vi "CheckStatus.vi"(0 "VISA resource name":refnum<visa-resource-name>, 3 "error in (no error)":errorcluster) -> (1 "Idle":bool, 4 "Target Reached":bool, 5 "VISA resource name out":refnum<visa-resource-name>, 6 "Infusing":bool, 7 "Withdrawing":bool, 8 "error out":errorcluster)   [LabVIEW 2018]
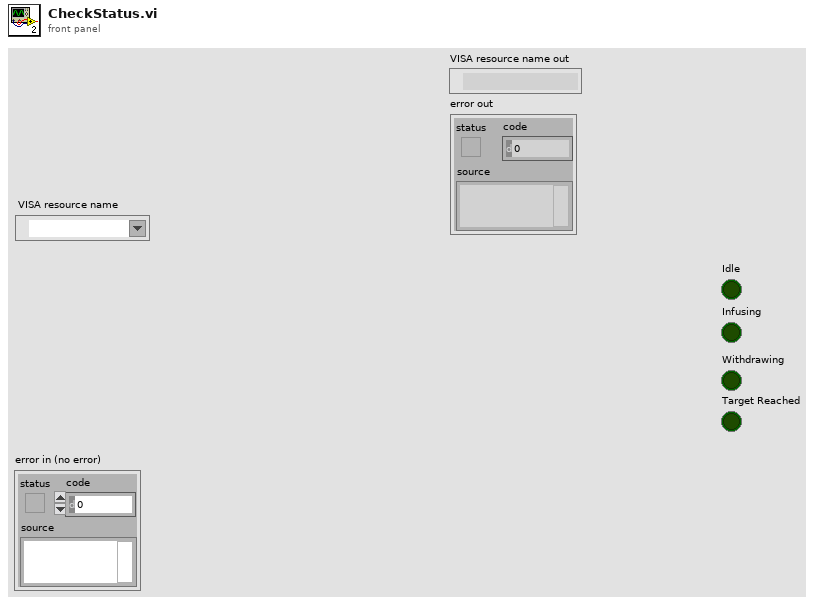
[diagram p1: front panel]
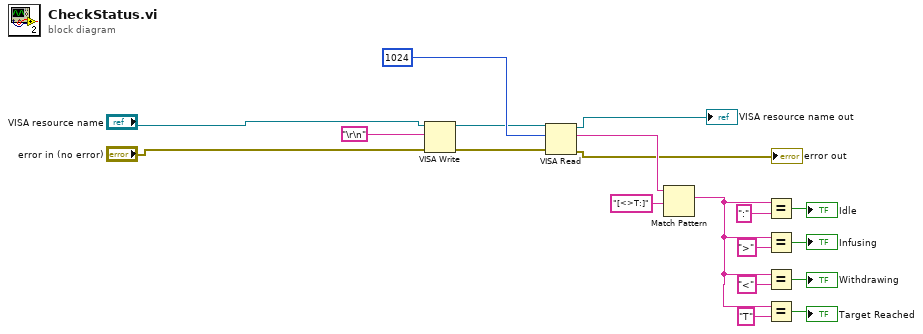
[diagram p0: block diagram]
diagram:
  n1 = VISA Write(VISA resource name="VISA resource name", write buffer="\r\n", error in (no error)="error in (no error)") -> (VISA resource name out=w7:refnum<visa-resource-name>, error out=w6:errorcluster)  [unwired: 1 out]
  n2 = VISA Read(VISA resource name=w7, byte count=u32 1024, error in (no error)=w6) -> (VISA resource name out=→"VISA resource name out":refnum<visa-resource-name>, read buffer=w17:string, error out=→"error out":errorcluster)  [unwired: 1 out]
  n3 = Match Pattern(string=w17, regular expression="[<>T:]") -> (match substring=w8:string)  [unwired: 1 in, 3 out]
  n4 = Equal?(x=w8, y=":") -> (x = y?=→"Idle":bool)
  n5 = Equal?(x=w8, y=">") -> (x = y?=→"Infusing":bool)
  n6 = Equal?(x=w8, y="<") -> (x = y?=→"Withdrawing":bool)
  n7 = Equal?(x=w8, y="T") -> (x = y?=→"Target Reached":bool)
